vi "Create Response.vi"(8 "error in (no error)":errorcluster, 11 "LV Server in":refnum<class "LV Server.lvclass">) -> (0 "error out":errorcluster, 2 "Response out":refnum<class "Response.lvclass">, 3 "LV Server out":refnum<class "LV Server.lvclass">)   [LabVIEW 2020, in "LV Server.lvclass"]
uses:
  LV Server.lvclass
  lv-http-util/HTTP Utils/Response/Response.lvclass
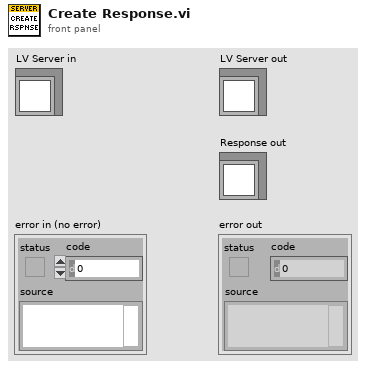
[diagram p1: front panel]
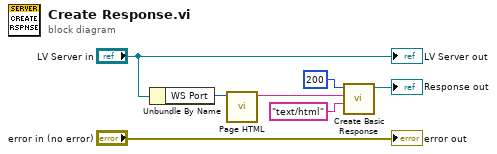
[diagram p0: block diagram]
diagram:
  n1 = Unbundle By Name("LV Server in") -> ("WS Port"=w1:u16)
  n2 = call "Page HTML.vi"("WS Port"=w1) -> ("Page HTML"=w4:string)  [unwired: 10 in]
  n3 = call "Create Basic Response.vi"("Content-Type (text/plain)"="text/html", "Payload"=w4, "Status Code"=u16 200) -> ("Response out"=→"Response out":refnum<class "Response.lvclass">)  [unwired: 7 in, 1 out]
  "error out" <- "error in (no error)"
  "LV Server out" <- "LV Server in"
